vi "treat request.vi"(8 "error in (no error)":errorcluster, 11 "S4GEI in":refnum<class "S4GEI.lvclass">) -> (0 "error out":errorcluster, 3 "S4GEI out":refnum<class "S4GEI.lvclass">)   [LabVIEW 2018, in "S4GEI.lvclass"]
uses:
  S4GEI.lvclass
  S4GEI.lvclass/S4GEI.ctl
  Channel GUI/Channel.lvclass/Channel.ctl
  State Machine/State Machine.lvclass
  Channel GUI/Channel.lvclass
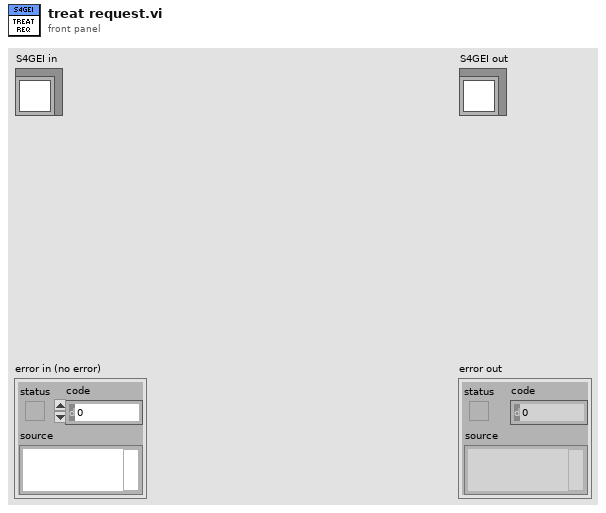
[diagram p1: front panel]
types:
  T1 = cluster{"State Machine.lvclass":refnum<class "State Machine.lvclass">, "RxTx.lvclass":refnum<class "RxTx.lvclass">, "Camera.lvclass":refnum<class "Camera.lvclass">, "Status RxTx.lvclass":refnum<class "RxTx.lvclass">}
  T2 = cluster{"Acquire":bool, "Stop Acquisition":bool, "Abort Acquisition":bool, "Pause acquisition":bool}
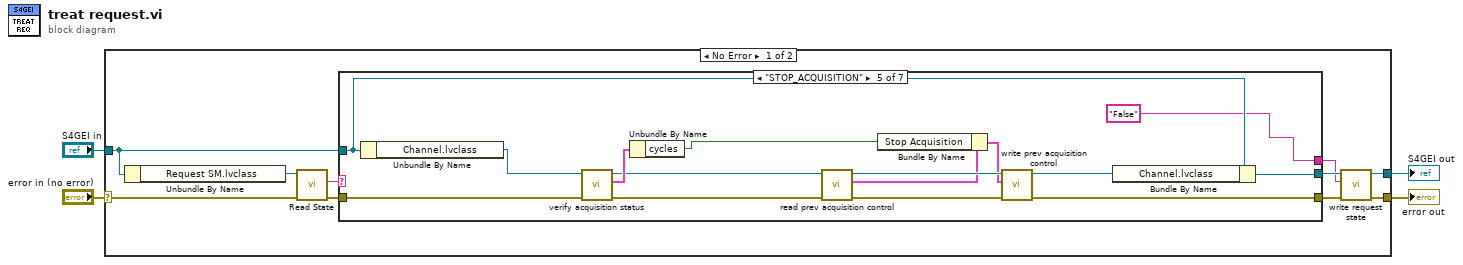
[diagram p0: block diagram]
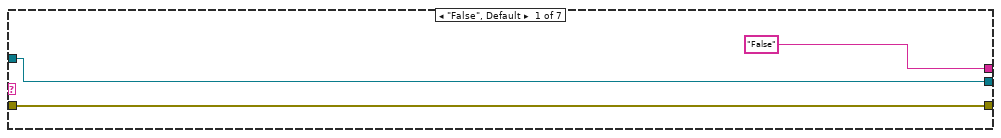
[diagram p2: hidden frame]
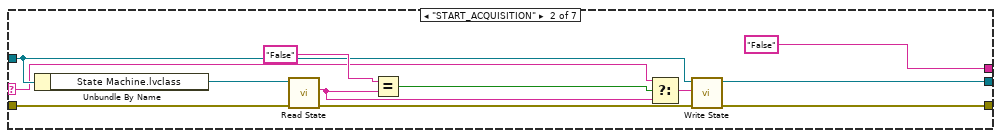
[diagram p3: hidden frame]
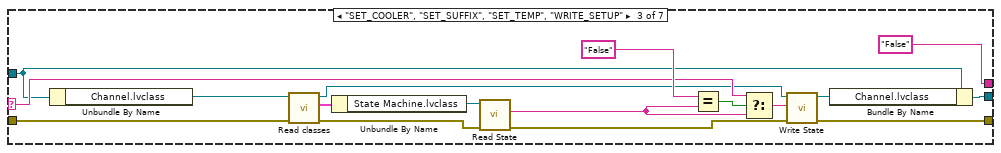
[diagram p4: hidden frame]
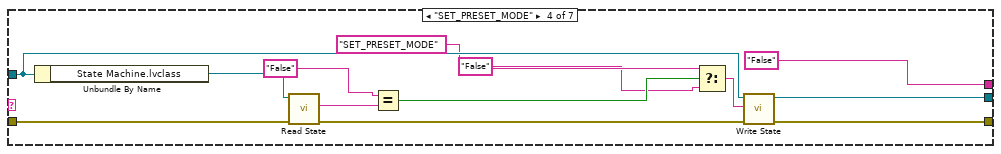
[diagram p5: hidden frame]
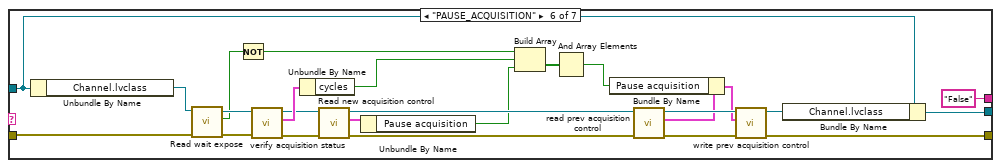
[diagram p6: hidden frame]
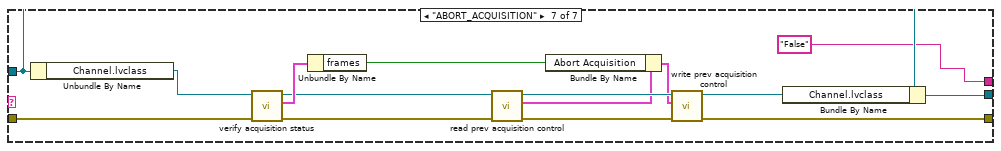
[diagram p7: hidden frame]
diagram:
  n1 = case shown="No Error" "error in (no error)" {
    selector: "error in (no error)" -> [w13 w116]
    tunnel: [w9 w116] -> w3
    tunnel: [w8 w115] -> w1
    tunnel: "S4GEI in" -> [w10 w115]
    frame No Error {
      n2 = Unbundle By Name(w10) -> ("Request SM.lvclass"=w14:refnum<class "State Machine.lvclass">)
      n3 = call-dynamic "Read State.vi"("error in (no error)"=w13, "State Machine in"=w14) -> ("error out"=w12:errorcluster, "State"=w11:string)  [unwired: 7 in, 1 out]
      n4 = case shown="\"STOP_ACQUISITION\"" w11 {
        selector: w11 -> [_ w19 w43 _ _ _ _]
        tunnel: w12 -> [w17 w28 w41 w57 w73 w83 w113]
        tunnel: w10 -> [w16 w25 w33 w54 w64 w93 w104]
        tunnel: [w17 w22 w31 w47 w65 w94 w105] -> w6
        tunnel: [w16 w21 w30 w48 w62 w91 w102] -> w7
        tunnel: ["False" ("x") "False" ("x") "False" ("x") "False" ("x") "False" ("x") "False" ("x") "False" ("x")] -> w5
        frame "False", Default {
        }
        frame "START_ACQUISITION" {
          n5 = Unbundle By Name(w25) -> ("State Machine.lvclass"=w29:refnum<class "State Machine.lvclass">)
          n6 = call-dynamic "Read State.vi"("error in (no error)"=w28, "State Machine in"=w29) -> ("error out"=w26:errorcluster, "State"=w18:string)  [unwired: 7 in, 1 out]
          n7 = Equal?(x="False", y=w18) -> (x = y?=w24:bool)
          n8 = Select(t=w19, s=w24, f=w18) -> (s? t:f=w23:string)
          n9 = call "Write State.vi"("error in (no error)"=w26, "State"=w23, "SPARC4_GEI in"=w25) -> ("error out"=w22:errorcluster, "SPARC4_GEI out"=w21:refnum<class "S4GEI.lvclass">)  [unwired: 7 in]
        }
        frame "SET_COOLER", "SET_SUFFIX", "SET_TEMP", "WRITE_SETUP" {
          n10 = Unbundle By Name(w33) -> ("Channel.lvclass"=w42:refnum<class "Channel.lvclass">)
          n11 = call-dynamic "Read classes.vi"("error in (no error)"=w41, "Channel in"=w42) -> ("error out"=w38:errorcluster, "classes"=w40:T1, "Channel out"=w36:refnum<class "Channel.lvclass">)  [unwired: 7 in]
          n12 = Unbundle By Name(w40) -> ("State Machine.lvclass"=w39:refnum<class "State Machine.lvclass">)
          n13 = call-dynamic "Read State.vi"("error in (no error)"=w38, "State Machine in"=w39) -> ("error out"=w35:errorcluster, "State"=w37:string)  [unwired: 7 in, 1 out]
          n14 = Equal?(x="False", y=w37) -> (x = y?=w45:bool)
          n15 = Select(t=w43, s=w45, f=w37) -> (s? t:f=w34:string)
          n16 = call "Write State.vi"("error in (no error)"=w35, "State"=w34, "Channel GEI in"=w36) -> ("error out"=w31:errorcluster, "Channel GEI out"=w32:refnum<class "Channel.lvclass">)  [unwired: 7 in]
          n17 = Bundle By Name(cluster=w33, "Channel.lvclass"=w32) -> (w30:refnum<class "S4GEI.lvclass">)
        }
        frame "SET_PRESET_MODE" {
          n18 = Unbundle By Name(w54) -> ("State Machine.lvclass"=w58:refnum<class "State Machine.lvclass">)
          n19 = call-dynamic "Read State.vi"("error in (no error)"=w57, "State Machine in"=w58) -> ("error out"=w53:errorcluster, "State"=w56:string)  [unwired: 7 in, 1 out]
          n20 = Equal?(x="False", y=w56) -> (x = y?=w52:bool)
          n21 = Select(t="SET_PRESET_MODE", s=w52, f="False") -> (s? t:f=w49:string)
          n22 = call "Write State.vi"("error in (no error)"=w53, "State"=w49, "SPARC4_GEI in"=w54) -> ("error out"=w47:errorcluster, "SPARC4_GEI out"=w48:refnum<class "S4GEI.lvclass">)  [unwired: 7 in]
        }
        frame "STOP_ACQUISITION" {
          n23 = Unbundle By Name(w64) -> ("Channel.lvclass"=w74:refnum<class "Channel.lvclass">)
          n24 = call "verify acquisition status.vi"("error in (no error)"=w73, "Channel in"=w74) -> ("error out"=w71:errorcluster, "acq status"=w72:cluster{"frames":bool, "cycles":bool}, "Channel out"=w68:refnum<class "Channel.lvclass">)  [unwired: 7 in]
          n25 = Unbundle By Name(w72) -> ("cycles"=w60:bool)
          n26 = call-dynamic "read prev acquisition control.vi"("error in (no error)"=w71, "Channel in"=w68) -> ("error out"=w69:errorcluster, "prev acquisition control"=w67:T2, "Channel out"=w70:refnum<class "Channel.lvclass">)  [unwired: 7 in]
          n27 = Bundle By Name(cluster=w67, "Stop Acquisition"=w60) -> (w66:T2)
          n28 = call-dynamic "write prev acquisition control.vi"("error in (no error)"=w69, "prev acquisition control"=w66, "Channel in"=w70) -> ("error out"=w65:errorcluster, "Channel out"=w63:refnum<class "Channel.lvclass">)  [unwired: 7 in]
          n29 = Bundle By Name(cluster=w64, "Channel.lvclass"=w63) -> (w62:refnum<class "S4GEI.lvclass">)
        }
        frame "PAUSE_ACQUISITION" {
          n30 = Unbundle By Name(w93) -> ("Channel.lvclass"=w84:refnum<class "Channel.lvclass">)
          n31 = call-dynamic "Read wait expose.vi"("error in (no error)"=w83, "Channel in"=w84) -> ("error out"=w82:errorcluster, "wait expose"=w75:bool, "Channel out"=w81:refnum<class "Channel.lvclass">)  [unwired: 7 in]
          n32 = Not(x=w75) -> (.not. x?=w76:bool)
          n33 = call "verify acquisition status.vi"("error in (no error)"=w82, "Channel in"=w81) -> ("error out"=w88:errorcluster, "acq status"=w99:cluster{"frames":bool, "cycles":bool}, "Channel out"=w89:refnum<class "Channel.lvclass">)  [unwired: 7 in]
          n34 = Unbundle By Name(w99) -> ("cycles"=w80:bool)
          n35 = call "Read new acquisition control.vi"("error in (no error)"=w88, "Channel in"=w89) -> ("error out"=w87:errorcluster, "new acquisition control"=w85:T2, "Channel out"=w86:refnum<class "Channel.lvclass">)  [unwired: 7 in]
          n36 = Unbundle By Name(w85) -> ("Pause acquisition"=w79:bool)
          n37 = Build Array(w76, w80, w79) -> (w78:bool[])
          n38 = And Array Elements(Boolean array=w78) -> (logical AND=w77:bool)
          n39 = call-dynamic "read prev acquisition control.vi"("error in (no error)"=w87, "Channel in"=w86) -> ("error out"=w97:errorcluster, "prev acquisition control"=w96:T2, "Channel out"=w98:refnum<class "Channel.lvclass">)  [unwired: 7 in]
          n40 = Bundle By Name(cluster=w96, "Pause acquisition"=w77) -> (w95:T2)
          n41 = call-dynamic "write prev acquisition control.vi"("error in (no error)"=w97, "prev acquisition control"=w95, "Channel in"=w98) -> ("error out"=w94:errorcluster, "Channel out"=w92:refnum<class "Channel.lvclass">)  [unwired: 7 in]
          n42 = Bundle By Name(cluster=w93, "Channel.lvclass"=w92) -> (w91:refnum<class "S4GEI.lvclass">)
        }
        frame "ABORT_ACQUISITION" {
          n43 = Unbundle By Name(w104) -> ("Channel.lvclass"=w114:refnum<class "Channel.lvclass">)
          n44 = call "verify acquisition status.vi"("error in (no error)"=w113, "Channel in"=w114) -> ("error out"=w111:errorcluster, "acq status"=w112:cluster{"frames":bool, "cycles":bool}, "Channel out"=w108:refnum<class "Channel.lvclass">)  [unwired: 7 in]
          n45 = Unbundle By Name(w112) -> ("frames"=w100:bool)
          n46 = call-dynamic "read prev acquisition control.vi"("error in (no error)"=w111, "Channel in"=w108) -> ("error out"=w109:errorcluster, "prev acquisition control"=w107:T2, "Channel out"=w110:refnum<class "Channel.lvclass">)  [unwired: 7 in]
          n47 = Bundle By Name(cluster=w107, "Abort Acquisition"=w100) -> (w106:T2)
          n48 = call-dynamic "write prev acquisition control.vi"("error in (no error)"=w109, "prev acquisition control"=w106, "Channel in"=w110) -> ("error out"=w105:errorcluster, "Channel out"=w103:refnum<class "Channel.lvclass">)  [unwired: 7 in]
          n49 = Bundle By Name(cluster=w104, "Channel.lvclass"=w103) -> (w102:refnum<class "S4GEI.lvclass">)
        }
      }
      n50 = call "write request state.vi"("error in (no error)"=w6, "State"=w5, "S4GEI in"=w7) -> ("error out"=w9:errorcluster, "S4GEI out"=w8:refnum<class "S4GEI.lvclass">)  [unwired: 7 in]
    }
    frame Error {
    }
  }
  "error out" <- w3
  "S4GEI out" <- w1
